vi "radius search byte.vi"(0 "index_ptr":u64, 1 "radius":sgl=1.0, 2 "max_nn":i32=1, 3 "Overwrite Lib Path":path, 5 "query points":u8[][](array[numeric]), 9 "flann_params":T1 {"algorithm" items=["FLANN_INDEX_LINEAR"=0, "FLANN_INDEX_KDTREE"=1, "FLANN_INDEX_KMEANS"=2, "FLANN_INDEX_COMPOSITE"=3, "FLANN_INDEX_KDTREE_SINGLE"=4, "FLANN_INDEX_HIERARCHICAL"=5, "FLANN_INDEX_LSH"=6, "FLANN_INDEX_SAVED"=254, "FLANN_INDEX_AUTOTUNED"=255]; "centers_init" items=["FLANN_CENTERS_RANDOM", "FLANN_CENTERS_GONZALES", "FLANN_CENTERS_KMEANSPP", "FLANN_CENTERS_GROUPWISE"]; "log_level" items=["FLANN_LOG_NONE", "FLANN_LOG_FATAL", "FLANN_LOG_ERROR", "FLANN_LOG_WARN", "FLANN_LOG_INFO", "FLANN_LOG_DEBUG"]}, 11 "error in (no error)":errorcluster) -> (4 "index_ptr out":u64, 6 "indices out":i32[][](array[numeric]), 8 "dists out":sgl[][](array[numeric]), 10 "flann_params":T1 {"algorithm" items=["FLANN_INDEX_LINEAR"=0, "FLANN_INDEX_KDTREE"=1, "FLANN_INDEX_KMEANS"=2, "FLANN_INDEX_COMPOSITE"=3, "FLANN_INDEX_KDTREE_SINGLE"=4, "FLANN_INDEX_HIERARCHICAL"=5, "FLANN_INDEX_LSH"=6, "FLANN_INDEX_SAVED"=254, "FLANN_INDEX_AUTOTUNED"=255]; "centers_init" items=["FLANN_CENTERS_RANDOM", "FLANN_CENTERS_GONZALES", "FLANN_CENTERS_KMEANSPP", "FLANN_CENTERS_GROUPWISE"]; "log_level" items=["FLANN_LOG_NONE", "FLANN_LOG_FATAL", "FLANN_LOG_ERROR", "FLANN_LOG_WARN", "FLANN_LOG_INFO", "FLANN_LOG_DEBUG"]}, 14 "N Found":i32[](array[numeric]), 15 "error out":errorcluster)   [LabVIEW 2020, in "KD Tree.lvlib"]
doc: "FLANN_EXPORT int flann_radius_search_double(flann_index_t index_ptr, \n double* query, \n int* indices, \n double* dists, \n int max_nn, \n float radius, \n struct FLANNParameters* flann_params);"
uses:
  KD Tree.lvlib
  Flann Params.ctl
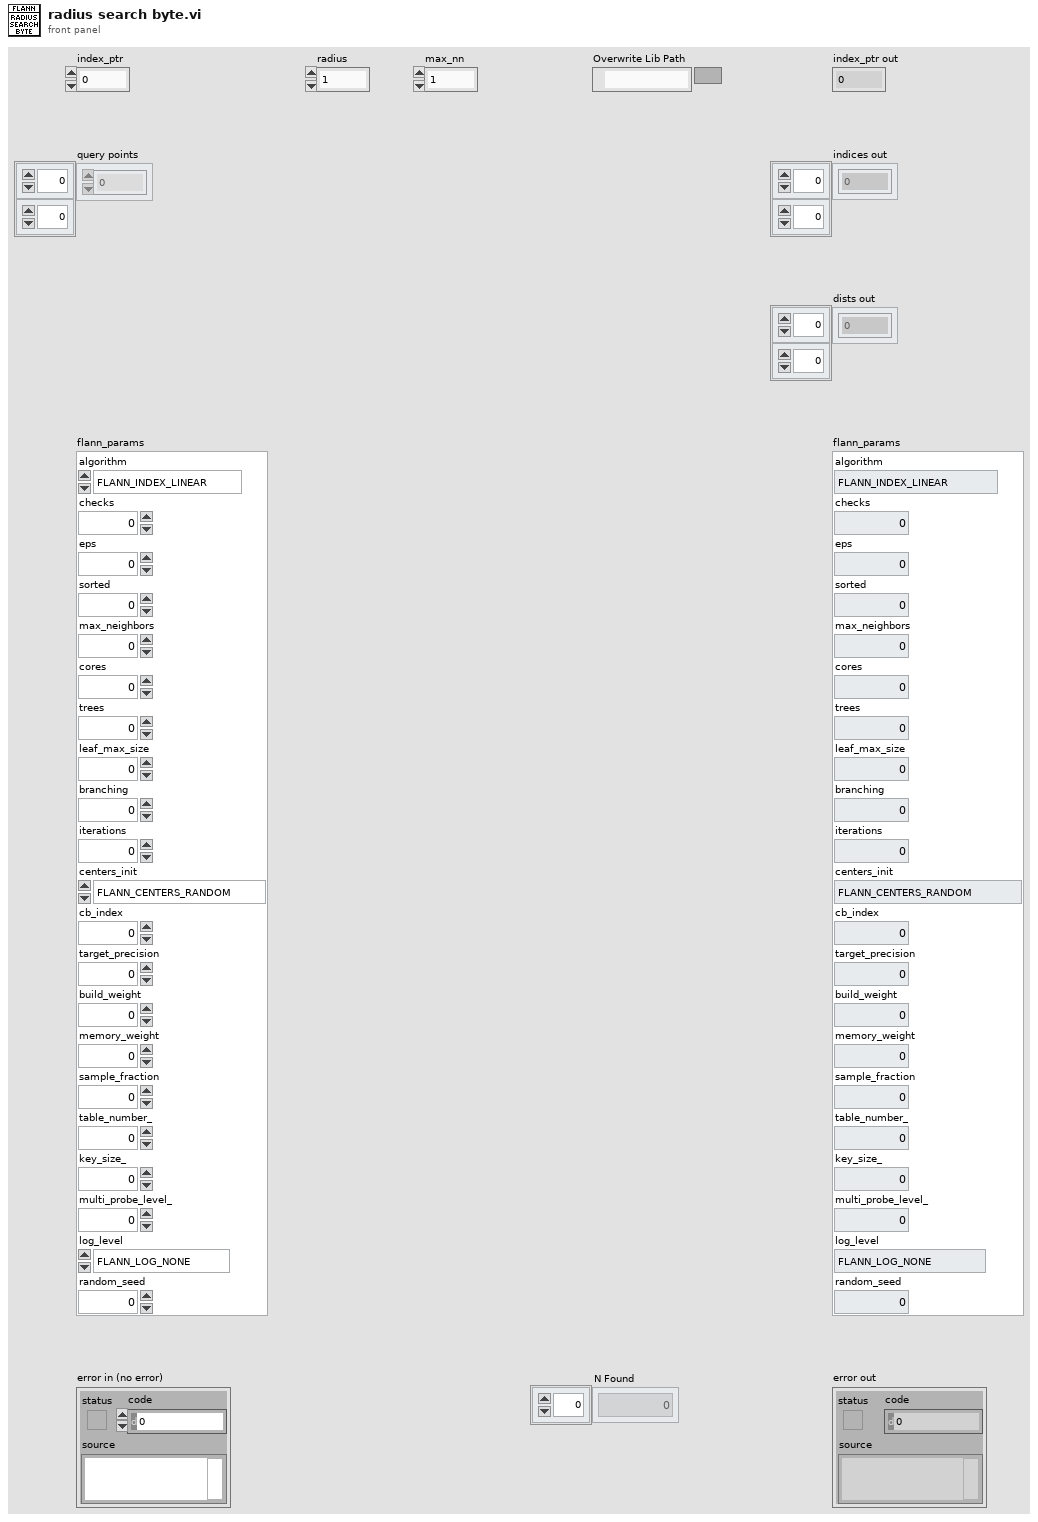
[diagram p1: front panel]
types:
  T1 = typedef "KD Tree.lvlib/Flann Params.ctl" = cluster{"algorithm":u32, "checks":i32, "eps":sgl, "sorted":i32, "max_neighbors":i32, "cores":i32, "trees":i32, "leaf_max_size":i32, "branching":i32, "iterations":i32, "centers_init":u32, "cb_index":sgl, "target_precision":sgl, "build_weight":sgl, "memory_weight":sgl, "sample_fraction":sgl, "table_number_":u32, "key_size_":u32, "multi_probe_level_":u32, "log_level":u32, "random_seed":i32}
  T2 = typedef "Semaphore RefNum" = refnum<k1>
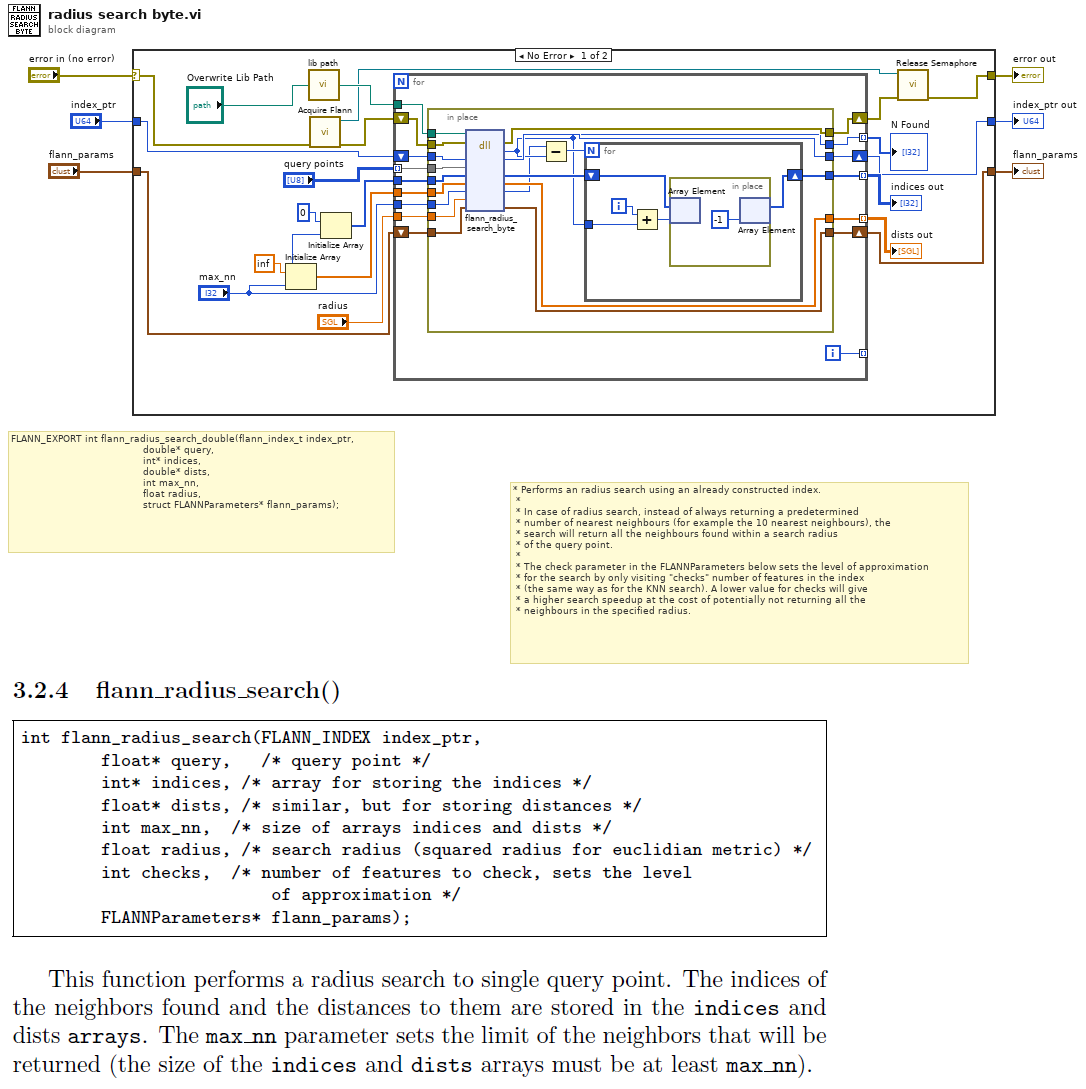
[diagram p0: block diagram]
diagram:
  # "* Performs an radius search using an already constructed index.\n *\n * In case of radius search, instead of always returning a predetermined\n * number of nearest neighbours (for example the 10 nearest neighbours), the\n * search will return all the neighbours found within a search radius\n * of the query point.\n *\n * The check parameter in the FLANNParameters below sets the level of approximation\n * for the search by only visiting \"checks\" number of features in the index\n * (the same way as for the KNN search). A lower value for checks will give\n * a higher search speedup at the cost of potentially not returning all the\n * neighbours in the specified radius."
  # "FLANN_EXPORT int flann_radius_search_double(flann_index_t index_ptr, \n                                            double* query, \n                                            int* indices, \n                                            double* dists, \n                                            int max_nn,  \n                                            float radius, \n                                            struct FLANNParameters* flann_params);"
  n1 = case shown="No Error" "error in (no error)" {
    selector: "error in (no error)" -> [w24 w70]
    tunnel: "flann_params" -> [w25 w69]
    tunnel: [w8 w70] -> w4
    tunnel: [w20 w69] -> w3
    tunnel: "index_ptr" -> [w19 w68]
    tunnel: [w18 w68] -> w1
    frame No Error {
      n2 = Initialize Array(sgl inf ("dists"), "max_nn") -> (w22:sgl[])
      n3 = call "lib path.vi"("Overwrite Lib Path"="Overwrite Lib Path") -> ("lib path"=w11:path)
      n4 = call "Acquire Flann.vi"("error in (no error)"=w24) -> ("error out"=w9:errorcluster, "semaphore"=w7:T2)  [unwired: 9 in]
      n5 = Initialize Array(0 ("indices"), "max_nn") -> (w23:i32[])
      n6 = for {
        tunnel: "radius" -> [w43]
        tunnel: "query points" -> [w38] mode=indexing
        shift-right: [w36] -> w20
        shift-left: w25 -> [w42]
        shift-right: [w32] -> w13
        shift-left: w9 -> [w41]
        shift-right: [w31] -> w18
        shift-left: w19 -> [w39]
        tunnel: w23 -> [w40]
        tunnel: [w33] -> w21 mode=indexing
        tunnel: w22 -> [w34]
        tunnel: [w35] -> w27 mode=indexing
        tunnel: "max_nn" -> [w37]
        tunnel: [w30] -> _ mode=indexing
        tunnel: [w29] -> w12 mode=indexing
        tunnel: w11 -> [w28]
        i -> [w30]
        n7 = in-place {
          in-place-border: w43 -> [w61]
          in-place-border: w42 -> [w60]
          in-place-border: w41 -> [w59]
          in-place-border: w40 -> [w58]
          in-place-border: w34 -> [w51]
          in-place-border: w39 -> [w57]
          in-place-border: w38 -> [w56]
          in-place-border: w37 -> [w55]
          in-place-border: [w53] -> w36
          in-place-border: [w52] -> w35
          in-place-border: [w50] -> w33
          in-place-border: [w49] -> w32
          in-place-border: [w48] -> w31
          in-place-border: [w46] -> w29
          in-place-border: w28 -> [w44]
          n8 = dll-call lib="E:/Labview/LV 2020/Libs/flann/flann.*" fn="flann_radius_search_byte"(path in=w44, error in=w59, "index_ptr"=w57, "query"=w56, "indices"=w58, "dists"=w51, "max_nn"=w55, "radius"=w61, "flann_params"=w60) -> (error out=w49:errorcluster, "return type"=w46:i32, "index_ptr"=w48:u64, "indices"=w54:i32[], "dists"=w52:sgl[], "max_nn"=w45:i32, "flann_params"=w53:T1)  [unwired: 3 in, 1 out]
          n9 = Subtract(x=w45, y=w46) -> (x-y=w47:i32)
          n10 = for {
            N: w47 -> [_]
            shift-right: [w65] -> w50
            shift-left: w54 -> [w66]
            tunnel: w46 -> [w62]
            i -> [w64]
            n11 = Add(x=w64, y=w62) -> (x+y=w63:i32)
            n12 = in-place {
              n13 = in-place-array #1(w66, w63) -> ()  [unwired: 1 out]
              n14 = in-place-array #1(-1) -> (w65:i32[])  [unwired: 1 out]
            }
          }
        }
      }
      "indices out" <- w21
      "dists out" <- w27
      "N Found" <- w12
      n15 = call <vilib>:"Release Semaphore.vi"("error in (no error)"=w13, "semaphore"=w7) -> ("error out"=w8:errorcluster)  [unwired: 4 in, 1 out]
    }
    frame Error {
    }
  }
  "error out" <- w4
  "flann_params" <- w3
  "index_ptr out" <- w1
